vi "ListExamples.vi"(10 "Folder":string) -> (0 "VI Paths":path[](array[path]), 1 "Paths":path[](array[path]), 2 "vis":string[](array[string]), 3 "filenames":string[](array[string]), 5 "folder names":string[](array[string]))   [LabVIEW 2022 SP3]
panel:
  out "String":string
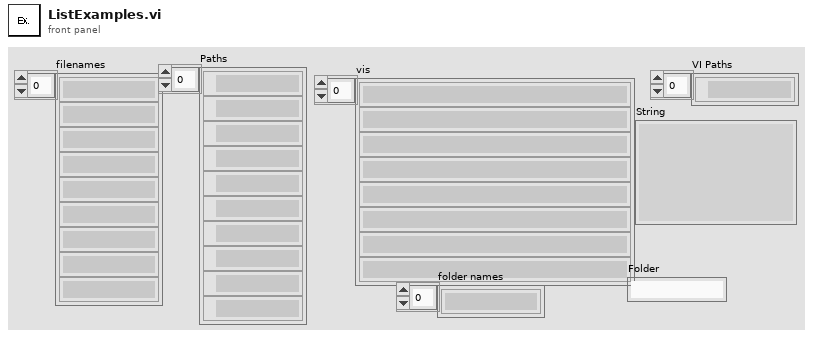
[diagram p1: front panel]
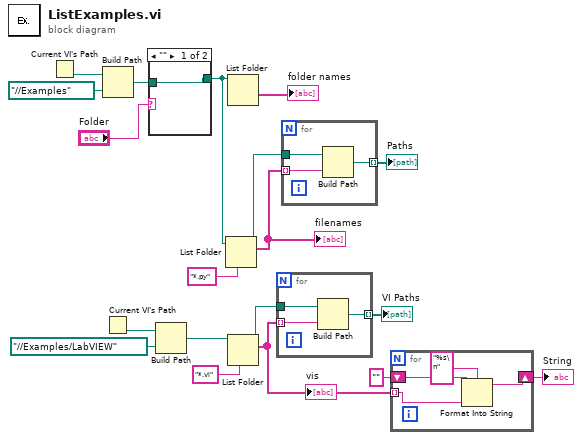
[diagram p0: block diagram]
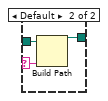
[diagram p2: hidden frame]
diagram:
  n1 = Current VI's Path() -> (path=w8:path)
  n2 = Build Path(base path=w8, name or relative path=path "../../Examples") -> (appended path=w6:path)
  n3 = Current VI's Path() -> (path=w14:path)
  n4 = case shown="\"\"" "Folder" {
    selector: "Folder" -> [_ w21]
    tunnel: w6 -> [w20 w23]
    tunnel: [w20 w22] -> w5
    frame "" {
    }
    frame Default {
      n5 = Build Path(base path=w23, name or relative path=w21) -> (appended path=w22:path)
    }
  }
  n6 = Build Path(base path=w14, name or relative path=path "../../Examples/LabVIEW") -> (appended path=w13:path)
  n7 = List Folder(path=w5, pattern="*.py") -> (path out=w18:path, filenames=w17:string[])  [unwired: 2 in, 2 out]
  "filenames" <- w17
  n8 = List Folder(path=w5) -> (folder names=→"folder names":string[])  [unwired: 3 in, 3 out]
  n9 = List Folder(path=w13, pattern="*.vi") -> (path out=w12:path, filenames=w3:string[])  [unwired: 2 in, 2 out]
  "vis" <- w3
  n10 = for {
    tunnel: w12 -> [w26]
    tunnel: w3 -> [w25] mode=indexing
    tunnel: [w24] -> w11 mode=indexing
    n11 = Build Path(base path=w26, name or relative path=w25) -> (appended path=w24:path)
  }
  "VI Paths" <- w11
  n12 = for {
    tunnel: w18 -> [w29]
    tunnel: w17 -> [w28] mode=indexing
    tunnel: [w27] -> w16 mode=indexing
    n13 = Build Path(base path=w29, name or relative path=w28) -> (appended path=w27:path)
  }
  "Paths" <- w16
  n14 = for {
    tunnel: w3 -> [w32] mode=indexing
    shift-right: [w31] -> w1
    shift-left: "" -> [w30]
    n15 = Format Into String(format string="%s\n", initial string=w30, w32) -> (resulting string=w31:string)  [unwired: 1 in, 1 out]
  }
  "String" <- w1
